vi "RAMP_save_path_definition_parameters.vi"(5 "error in":errorcluster, 6 "Sample name":string, 8 "Path to the saving folder":path) -> (0 "error out":errorcluster, 3 "Z_position_file path":path, 4 "Acquisition_parameters path":path)   [LabVIEW 2015]
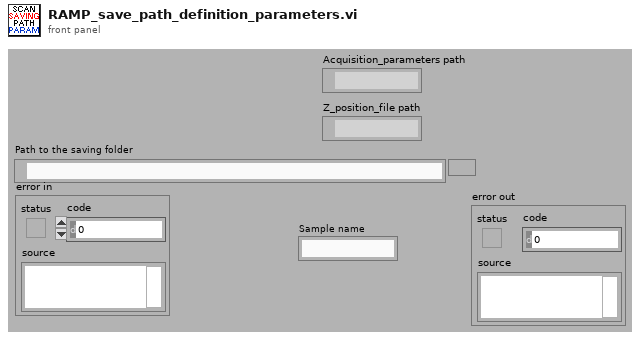
[diagram p1: front panel]
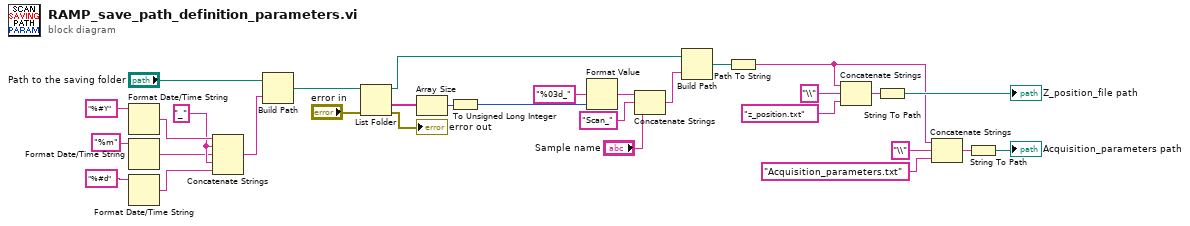
[diagram p0: block diagram]
diagram:
  w29 = "_" ("string")
  n1 = Format Date/Time String(time format string (%c)="%#Y") -> (date/time string=w30:string)  [unwired: 2 in]
  n2 = Format Date/Time String(time format string (%c)="%m") -> (date/time string=w26:string)  [unwired: 2 in]
  n3 = Format Date/Time String(time format string (%c)="%#d") -> (date/time string=w25:string)  [unwired: 2 in]
  n4 = Concatenate Strings(w30, w29, w26, w29, w25) -> (w23:string)
  n5 = Build Path(base path="Path to the saving folder", name or relative path=w23) -> (appended path=w4:path)
  n6 = List Folder(path=w4, error in="error in") -> (path out=w22:path, folder names=w5:string[], error out=→"error out":errorcluster)  [unwired: 2 in, 1 out]
  n7 = Array Size(array=w5) -> (size(s)=w6:i32)
  n8 = To Unsigned Long Integer(number=w6) -> (unsigned 32bit integer=w14:u32)
  n9 = Format Value(format string="%03d_" ("string (\"\")"), value (0)=w14) -> (output string=w13:string)  [unwired: 1 in]
  n10 = Concatenate Strings(w13, "Scan_" ("string"), "Sample name") -> (w11:string)
  n11 = Build Path(base path=w22, name or relative path=w11) -> (appended path=w1:path)
  n12 = Path To String(path=w1) -> (string=w8:string)
  n13 = Concatenate Strings(w8, "\\" ("string"), "z_position.txt" ("string")) -> (w20:string)
  n14 = String To Path(string=w20) -> (path=→"Z_position_file path":path)
  n15 = Concatenate Strings(w8, "\\" ("string"), "Acquisition_parameters.txt" ("string")) -> (w18:string)
  n16 = String To Path(string=w18) -> (path=→"Acquisition_parameters path":path)
